vi "Write Calibration.vi"(8 "error in (no error)":errorcluster, 10 "Calibration":T1={"scale"=1.0, "offset"=0.0}, 11 "FSR in":refnum<class "FSR.lvclass">) -> (0 "error out":errorcluster, 3 "FSR out":refnum<class "FSR.lvclass">)   [LabVIEW 2013, in "SGDV_Ctrl_v13_lib.lvlib" / "FSR.lvclass"]
uses:
  FSR.lvclass
  Common/Calibration.ctl
  FSR.lvclass/FSR.ctl
  SGDV_Ctrl_v13_lib.lvlib
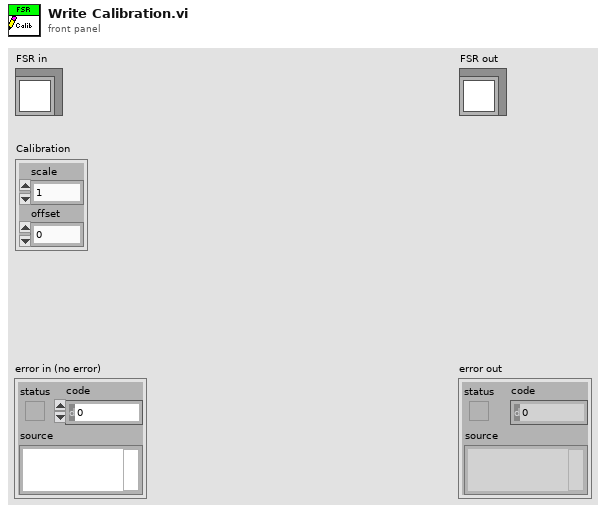
[diagram p1: front panel]
types:
  T1 = typedef "SGDV_Ctrl_v13_lib.lvlib/Calibration.ctl" = cluster{"scale":dbl, "offset":dbl}
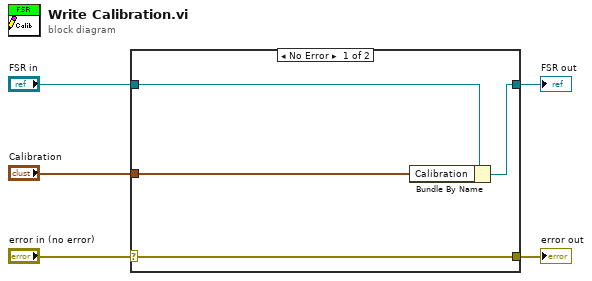
[diagram p0: block diagram]
diagram:
  n1 = case shown="No Error" "error in (no error)" {
    selector: "error in (no error)" -> [w9 w10]
    tunnel: [w9 w10] -> w4
    tunnel: [w7 w11] -> w2
    tunnel: "FSR in" -> [w8 w11]
    tunnel: "Calibration" -> [w6 _]
    frame No Error {
      n2 = Bundle By Name(cluster=w8, "Calibration"=w6) -> (w7:refnum<class "FSR.lvclass">)
    }
    frame Error {
    }
  }
  "error out" <- w4
  "FSR out" <- w2
